vi "Append ID.vi"(10 "name":string, 11 "initial id string (\"\")":string) -> (3 "appended id string":string)   [LabVIEW 2017, in "DSF Core.lvlib" / "Configuration Session.lvclass"]
uses:
  Configuration Session.lvclass
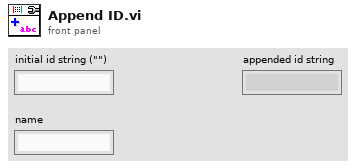
[diagram p1: front panel]
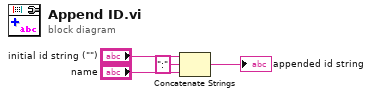
[diagram p0: block diagram]
diagram:
  n1 = Concatenate Strings("initial id string (\"\")", ":" ("string"), "name") -> (→"appended id string":string)
